vi "2012_07_10 read data.vi"(0 "MC Power":refnum<k21>, 1 "Motor Power":refnum<k21>, 11 "Error In":errorcluster) -> (3 "Motor Power Out":refnum<k21>, 4 "MC Power Out":refnum<k21>, 6 "Motor Power Data":waveform(dbl)[](array[waveform]), 8 "MC Power Data":waveform(dbl)[](array[waveform]), 15 "error out":errorcluster)   [LabVIEW 2011]
uses:
  <vilib>/DAQmx/read.llb/DAQmx Read (Analog 1D Wfm NChan NSamp).vi
  <vilib>/DAQmx/miscellaneous.llb/DAQmx Fill In Error Info.vi
panel:
  # "MC1"
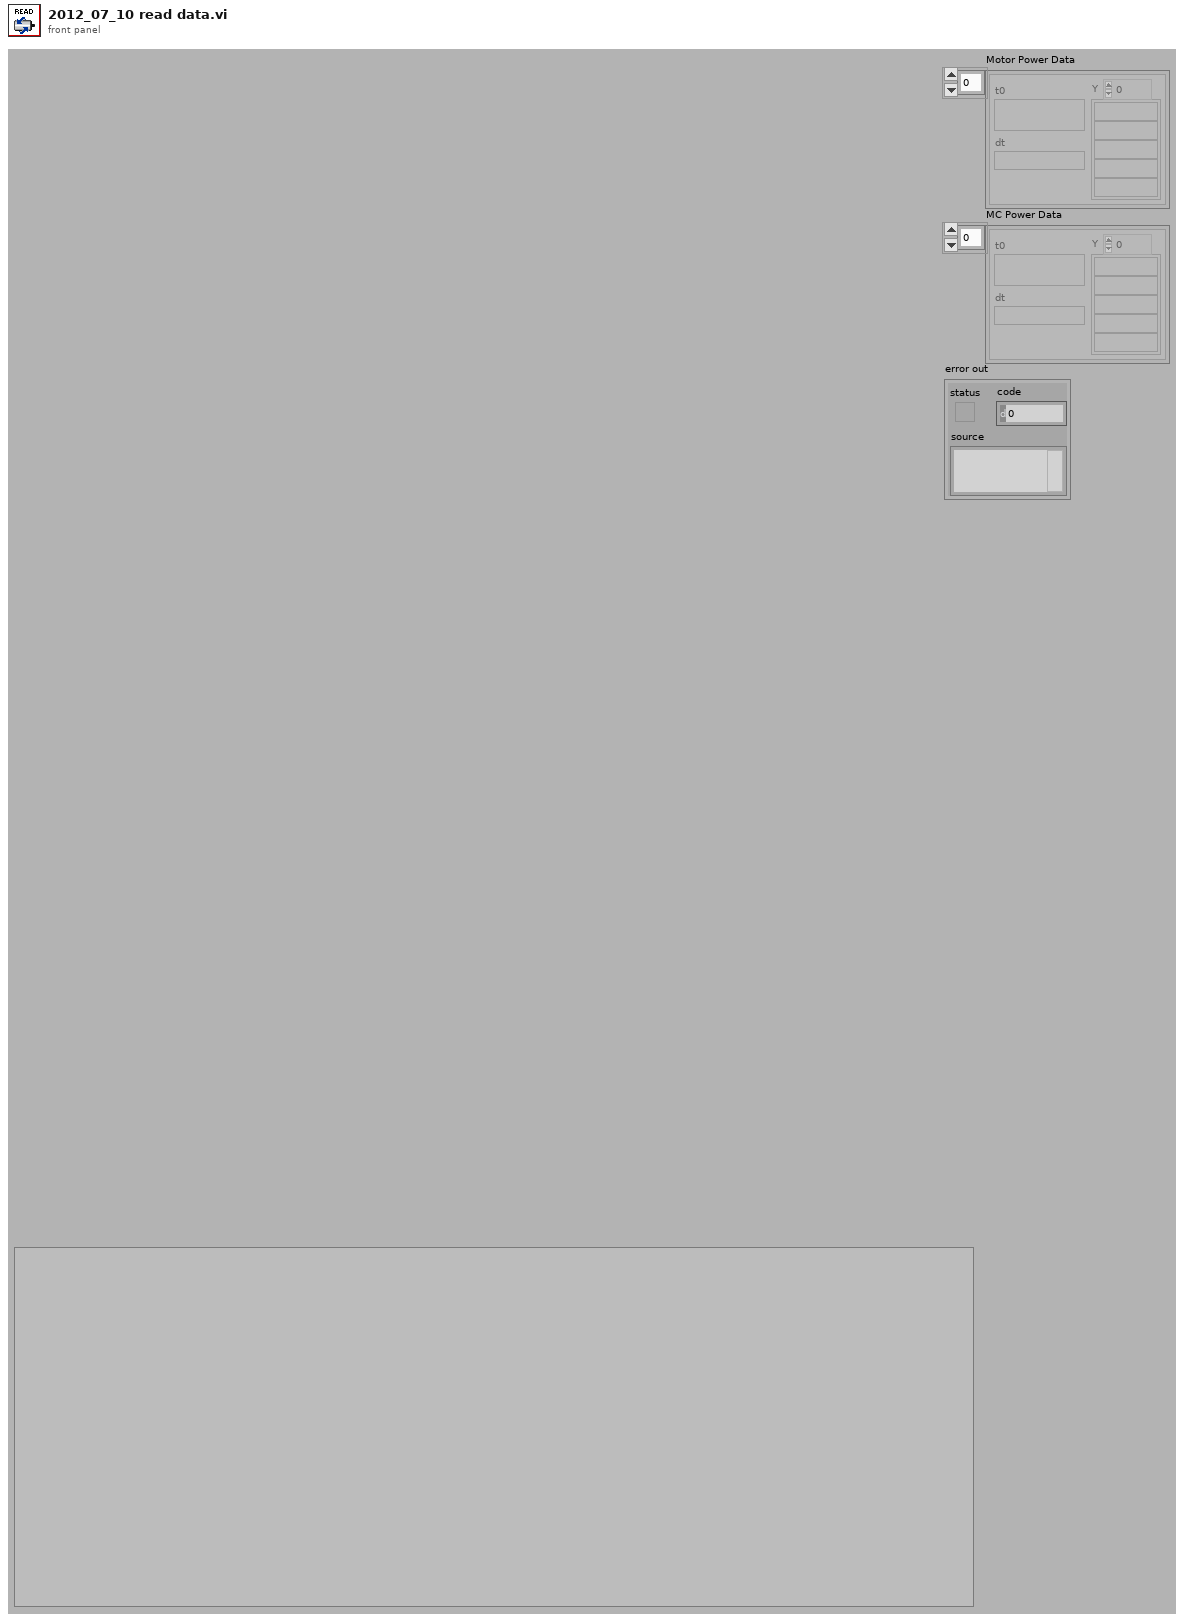
[diagram p1: front panel]
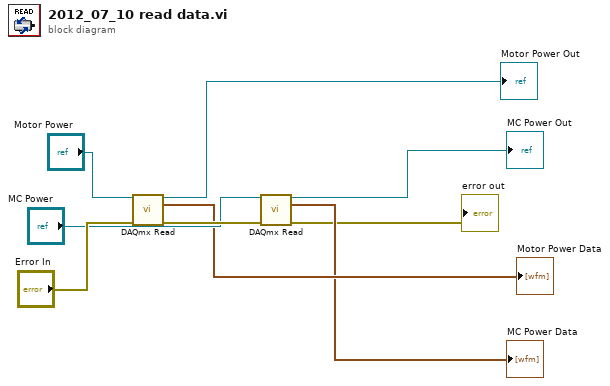
[diagram p0: block diagram]
diagram:
  n1 = call-poly <vilib>:"DAQmx Read.vi"("task/channels in"="Motor Power", "error in"="Error In") -> ("task out"=→"Motor Power Out":refnum<k21>, "data"=→"Motor Power Data":waveform(dbl)[], "error out"=w6:errorcluster)  [unwired: 11 in]
  n2 = call-poly <vilib>:"DAQmx Read.vi"("task/channels in"="MC Power", "error in"=w6) -> ("task out"=→"MC Power Out":refnum<k21>, "data"=→"MC Power Data":waveform(dbl)[], "error out"=→"error out":errorcluster)  [unwired: 11 in]
